vi "Read Counter Unit.vi"(8 "error in":errorcluster, 10 "Device":T1) -> (0 "error out":errorcluster)   [LabVIEW 2024, in "FlexiFlowInterface.lvlib"]
doc: "Reads the counter unit.\n_____\nCreated using DQMH Event Scripter 7.0.1.1316."
uses:
  FlexiFlowInterface.lvlib
  FlexiFlowDevice--enum.ctl
  Read Counter Unit Argument--cluster.ctl
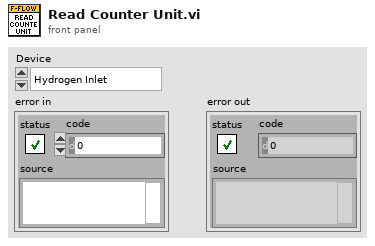
[diagram p1: front panel]
types:
  T1 = typedef "FlexiFlowInterface.lvlib/FlexiFlowDevice--enum.ctl" = enum16{"Hydrogen Inlet", "Nitrogen Inlet", "Cathode Outlet", "Anode Outlet"}
  T2 = typedef "FlexiFlowInterface.lvlib/Read Counter Unit Argument--cluster.ctl" = cluster{"Device":T1}
  T3 = typedef "FlexiFlowInterface.lvlib/Request Events--cluster.ctl" = cluster{"Stop Module":refnum<user-event>, "Show Panel":refnum<user-event>, "Hide Panel":refnum<user-event>, "Get Module Execution Status":refnum<user-event>, "Show Diagram":refnum<user-event>, "Change Panel":refnum<user-event>, "Private":cluster{"Start Modbus Polling Helper Loop":refnum<user-event>, "Sleep Modbus Polling Helper Loop":refnum<user-event>, "Wake Connection Helper Loop":refnum<user-event>, "Sleep Connection Helper Loop":refnum<user-event>}, "Initialise Modbus Connections":refnum<user-event>, "Read Fmeasure":refnum<user-event>, "Set Modbus Configuration":refnum<user-event>, "Wink Devices":refnum<user-event>, "Read All FlexiFlow Device States":refnum<user-event>, "Wink Device":refnum<user-event>, "Set Control Function":refnum<user-event>, "Set Flow Setpoint":refnum<user-event>, "Set Backpressure Setpoint":refnum<user-event>, "Set Forward Pressure SP":refnum<user-event>, "Set Capacity Unit":refnum<user-event>, "Set Flow Capacity Unit":refnum<user-event>, "Set Setpoint Slope":refnum<user-event>, "Set Counter Settings":refnum<user-event>, "Reset All Device Counters":refnum<user-event>, "Read Device User Tag":refnum<user-event>, "Set Device User Tag":refnum<user-event>, "Read Counter Unit":refnum<user-event>, "Set Control Mode":refnum<user-event>, "Get Device Configuration":refnum<user-event>}
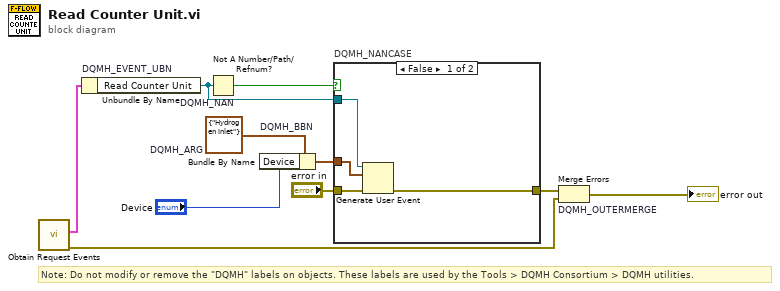
[diagram p0: block diagram]
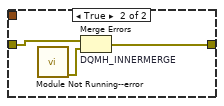
[diagram p2: hidden frame]
diagram:
  w4 = T2 {"Device"=enum."Hydrogen Inlet"}  # DQMH_ARG
  # "Note: Do not modify or remove the \"DQMH\" labels on objects. These labels are used by the Tools > DQMH Consortium > DQMH utilities."
  n1 = call "Obtain Request Events.vi"() -> ("error out"=w3:errorcluster, "FlexiFlowInterface Request Events"=w2:T3)  [unwired: 10 in]
  n2 = Unbundle By Name "DQMH_EVENT_UBN"(w2) -> ("Read Counter Unit"=w6:refnum<user-event>)
  n3 = Not A Number/Path/Refnum? "DQMH_NAN"(number/path/refnum=w6) -> (NaN/Path/Refnum?=w7:bool)
  n4 = Bundle By Name "DQMH_BBN"(cluster=w4, "Device"="Device") -> (w8:T2)
  n5 = case "DQMH_NANCASE" shown="False" w7 {
    tunnel: "error in" -> [w14 w17]
    tunnel: [w13 w16] -> w5
    tunnel: w6 -> [w12 _]
    tunnel: w8 -> [w11 _]
    frame False {
      n6 = Generate User Event(user event=w12, event data cluster=w11, error in=w14) -> (error out=w13:errorcluster)  [unwired: 1 in, 1 out]
    }
    frame True {
      n7 = call "Module Not Running--error.vi"() -> ("error out"=w15:errorcluster)  [unwired: 11 in]
      n8 = Merge Errors "DQMH_INNERMERGE"(w17, w15) -> (w16:errorcluster)
    }
  }
  n9 = Merge Errors "DQMH_OUTERMERGE"(w5, w3) -> (→"error out":errorcluster)
